vi "SetupDefault.vi"(8 "error in (no error)":errorcluster, 10 "Alias":string, 11 "PSU_N87 in":refnum<class "PSU_N67.lvclass">) -> (0 "error out":errorcluster, 3 "PSU_N87 out":refnum<class "PSU_N67.lvclass">)   [LabVIEW 2014, in "PSU_N67.lvclass"]
uses:
  PSU_N67.lvclass
  PSU_N67.lvclass/PSU_N67.ctl
  data/Agilent N6700 Series.lvlib
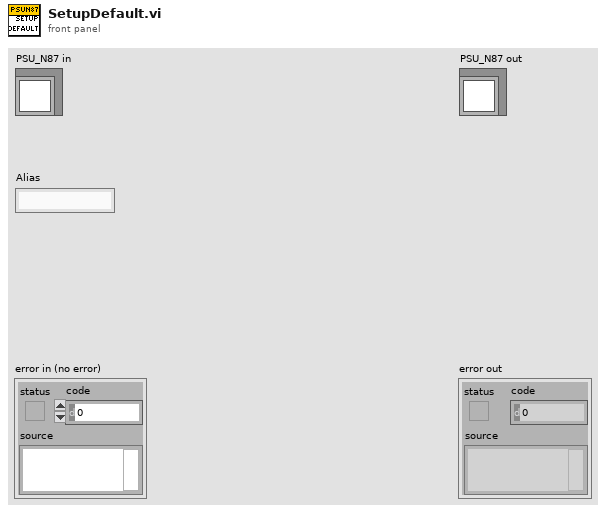
[diagram p1: front panel]
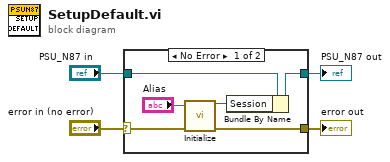
[diagram p0: block diagram]
diagram:
  n1 = case shown="No Error" "error in (no error)" {
    selector: "error in (no error)" -> [w5 w11]
    tunnel: "PSU_N87 in" -> [w10 w12]
    tunnel: [w9 w12] -> w2
    tunnel: [w6 w11] -> w1
    frame No Error {
      n2 = call "Initialize.vi"("VISA resource name"="Alias", "error in (no error)"=w5) -> ("VISA resource name out"=w7:refnum<visa-resource-name>, "error out"=w6:errorcluster)  [unwired: 12 in]
      n3 = Bundle By Name(cluster=w10, "Session"=w7) -> (w9:refnum<class "PSU_N67.lvclass">)
    }
    frame Error {
    }
  }
  "error out" <- w1
  "PSU_N87 out" <- w2
